vi "Open Plotter Session.vi"(8 "error in (no error)":errorcluster, 11 "PythonPlotter in":refnum<class "PythonPlotter.lvclass">) -> (0 "error out":errorcluster, 3 "PythonPlotter out":refnum<class "PythonPlotter.lvclass">)   [LabVIEW 2024, in "PythonPlotter.lvclass"]
uses:
  PythonPlotter.lvclass
  PythonPlotter.lvclass/PythonPlotter.ctl
  <vilib>/Python/Open Venv Python Session.vi
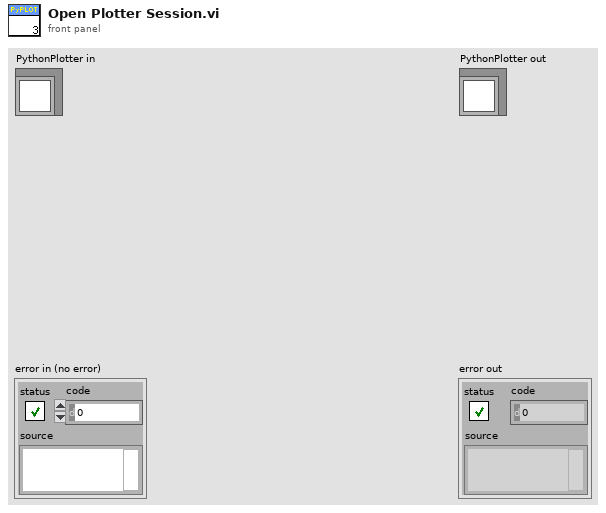
[diagram p1: front panel]
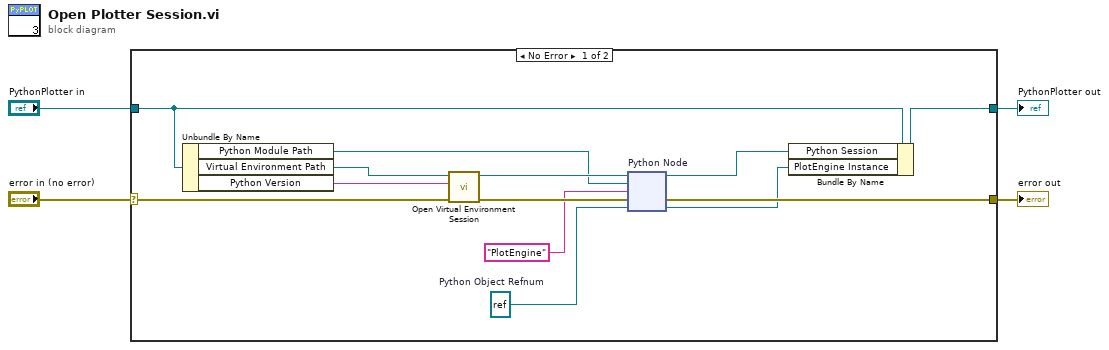
[diagram p0: block diagram]
diagram:
  n1 = case shown="No Error" "error in (no error)" {
    selector: "error in (no error)" -> [w12 w19]
    tunnel: [w13 w19] -> w3
    tunnel: [w7 w18] -> w1
    tunnel: "PythonPlotter in" -> [w11 w18]
    frame No Error {
      w14 = refnum<k38> refnum  # Python Object Refnum
      n2 = Unbundle By Name(w11) -> ("Python Module Path"=w8:path, "Virtual Environment Path"=w10:path, "Python Version"=w9:string)
      n3 = call-poly <vilib>:"Open Virtual Environment Session.vi"("error in (no error)"=w12, "Python version"=w9, "Env path"=w10) -> ("error out"=w16:errorcluster, "session out"=w17:refnum<k35>)  [unwired: 7 in]
      n4 = node "Python Node"(w17, w8, "PlotEngine" ("function name"), w16, w14) -> (w6:refnum<k35>, w13:errorcluster, w5:refnum<k38>)  [unwired: 2 out]
      n5 = Bundle By Name(cluster=w11, "Python Session"=w6, "PlotEngine Instance"=w5) -> (w7:refnum<class "PythonPlotter.lvclass">)
    }
    frame Error {
    }
  }
  "error out" <- w3
  "PythonPlotter out" <- w1
